vi "Vision 배열 분리.vi"(5 "행렬":T1) -> (0 "Vision Distance (m)":dbl[](array[numeric]), 1 "X":dbl[][](array[numeric]), 2 "Vision Angle (rad)":dbl[](array[numeric]))   [LabVIEW 2016]
uses:
  <vilib>/Analysis/Matrix/Datatypes/RealMatrix.ctl
  <vilib>/imath/engines/lvmath2/RunTimeEngine/Managers/WorkSpace/UID Generator.vi
  <vilib>/imath/engines/lvmath2/RunTimeEngine/BuiltInFunctions/deg_to_rad/NIMS_deg_to_rad.vi
  <instcachedir>/0/NIMS_deg_to_rad_4A81D684CE8D4DD79924F5AB74D756E1.lvgen/NIMS_deg_to_rad_4A81D684CE8D4DD79924F5AB74D756E1_002.vi
  <vilib>/imath/engines/lvmath2/RunTimeEngine/RunTimeType/NIMS_RunTimeType_From StrictType (excl LVString).vi
  <instcachedir>/0/NIMS_RunTimeType_From StrictType (excl LVString)_BBF44FB49F834B71AF7A14CCEDF8BECD.lvgen/NIMS_RunTimeType_From StrictType (excl LVString)_BBF44FB49F834B71AF7A14CCEDF8BECD_000.vi
  <vilib>/imath/engines/lvmath2/RunTimeEngine/LocalVariableDefStatement/MC_LocalVariableDefStatement_Display.vi
  <vilib>/imath/engines/lvmath2/RunTimeEngine/MatrixToken/NIMS_MatrixToken_RV_RV.vi
  <instcachedir>/0/NIMS_MatrixToken_RV_RV_41289AEE7DB340EFBB9CA44FA48DA89B.lvgen/NIMS_MatrixToken_RV_RV_41289AEE7DB340EFBB9CA44FA48DA89B_002.vi
  <vilib>/imathl/engines/lvmath/Functions/Error Handling/Create Error.vi
  <vilib>/imath/engines/lvmath2/RunTimeEngine/Managers/SymbolTable/Clear UID.vi
  <vilib>/imath/engines/lvmath2/RunTimeEngine/NodeEndStatement/NIMS_NodeEndStatement_Output.vi
  <instcachedir>/0/NIMS_NodeEndStatement_Output_53EC0D466D134D7ABD903AC30B43404B.lvgen/NIMS_NodeEndStatement_Output_53EC0D466D134D7ABD903AC30B43404B_002.vi
  <instcachedir>/0/NIMS_NodeEndStatement_Output_53EC0D466D134D7ABD903AC30B43404B.lvgen/NIMS_NodeEndStatement_Output_53EC0D466D134D7ABD903AC30B43404B_005.vi
  <vilib>/imath/engines/lvmath2/RunTimeEngine/ErrorHandling/NIMS_Finalize Error.vi
  <vilib>/imath/engines/lvmath2/RunTimeEngine/Managers/SymbolTable/NIMS_WorkSpace.lvlib
  <vilib>/Analysis/Matrix/NI_Matrix.lvlib
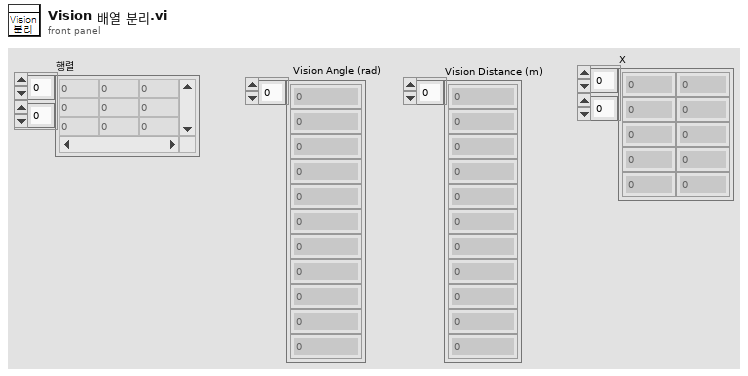
[diagram p1: front panel]
types:
  T1 = typedef "NI_Matrix.lvlib/RealMatrix.ctl" = dbl[][]
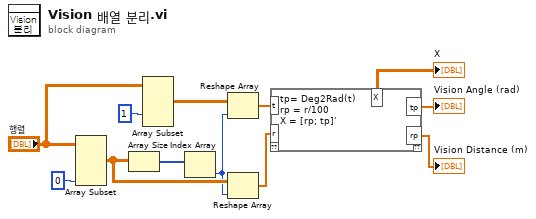
[diagram p0: block diagram]
diagram:
  n1 = Array Subset(array="행렬", length (col)=0 ("행 1")) -> (w10:T1)  [unwired: 3 in]
  n2 = Array Size(array=w10) -> (size(s)=w8:i32[])
  n3 = Array Subset(array="행렬", index (col)=1 ("열 1")) -> (w9:T1)  [unwired: 3 in]
  n4 = Index Array(array=w8) -> (element=w7:i32)  [unwired: 1 in]
  n5 = Reshape Array(w9, w7) -> (w5:dbl[])
  n6 = Reshape Array(w10, w7) -> (w2:dbl[])
  n7 = mathscript code="tp= Deg2Rad(t)\nrp = r/100\nX = [rp; tp]'"("t"=w5, "r"=w2) -> ("tp"=→"Vision Angle (rad)":dbl[], "rp"=→"Vision Distance (m)":dbl[], "X"=→"X":dbl[][])  [unwired: 1 in, 1 out]
